vi "Teleop.vi"(10 "Match Info":T1={"Autonomous Elapsed Seconds"=0.0, "TeleOp Elapsed Seconds"=0.0, "Disabled Elapsed Seconds"=0.0, "Visited Autonomous"=FALSE, "Visited TeleOp"=FALSE, "Visited Disabled"=FALSE, "Autonomous Settings"={"Autonomous Style"=enum."Independent", "VI Refnum"=refnum}}, 11 "Call Context":T2) -> ()   [LabVIEW 2020]
doc: "This VI is called for each TeleOp packet received from the DS where the robot is not disabled. It is often used to read from the joysticks and update I/O or to update setpoints for timed control loops. It should complete and return within 20 milliseconds or it may miss DS packets."
uses:
  <vilib>/Rock Robotics/WPI/DriverStation/WPI_DriverStationDerivedRobotMode.ctl
  <vilib>/Rock Robotics/WPI/DriverStation/WPI_DriverStationMatch Info.ctl
  <vilib>/Rock Robotics/WPI/ThirdParty/Phoenix-LabVIEW/Motor Controller/Controls/CTRE_Phoenix_MotorControl_ControlMode.ctl
  <vilib>/Rock Robotics/WPI/Solenoid/WPI_SolenoidValue.ctl
  <vilib>/Rock Robotics/WPI/Utilities/WPI_GetSetVariantRefNum.vi
  <vilib>/Rock Robotics/Network Tables/NT Write Boolean Array.vi
  <vilib>/Rock Robotics/Network Tables/NT Write Numeric Array.vi
  <vilib>/Rock Robotics/Network Tables/NT Read Boolean.vi
  <vilib>/Rock Robotics/WPI/Solenoid/WPI_SolenoidSetEnum.vi
  Lime.vi
  <vilib>/Rock Robotics/WPI/RobotDrive/WPI_RobotDriveMecanumDrive_Cartesian.vi
panel:
  in  "Numeric":dbl=-0.7 format="%#_13g"
  in  "Auger Speed":dbl=-0.8
  out "Present Text":string
  in  "Total Time":dbl=0.9 format="%#_13g"
  in  "Time Low":dbl=0.6 format="%#_13g"
  in  "Slowmode Speed":dbl=0.33
  out "Compressor Running":bool
  out "Enabled":bool
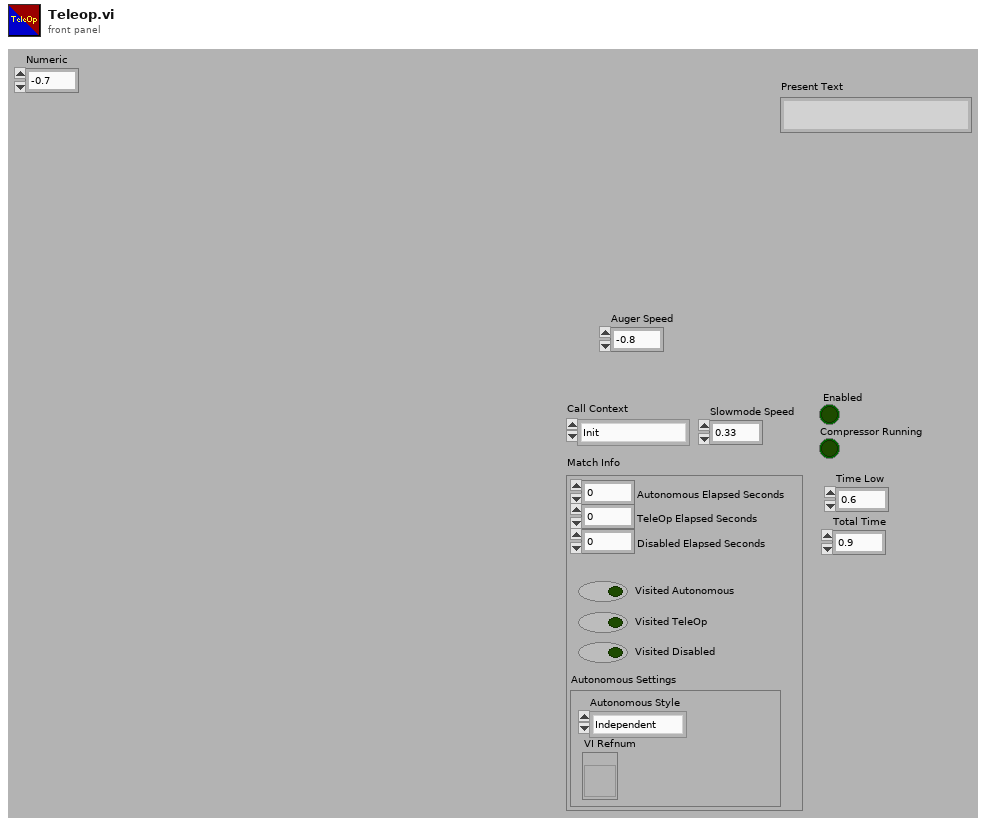
[diagram p1: front panel]
types:
  T1 = typedef "WPI_DriverStationMatch Info.ctl" = cluster{"Autonomous Elapsed Seconds":dbl, "TeleOp Elapsed Seconds":dbl, "Disabled Elapsed Seconds":dbl, "Visited Autonomous":bool, "Visited TeleOp":bool, "Visited Disabled":bool, "Autonomous Settings":cluster{"Autonomous Style":enum16{"Iterative", "Independent"}, "VI Refnum":refnum<vi>}}
  T2 = typedef "WPI_DriverStationDerivedRobotMode.ctl" = enum16{"Init", "Execute", "Stop"}
  T3 = typedef "CTRE_Phoenix_MotorControl_ControlMode.ctl" = u16
  T4 = typedef "WPI_JoystickDevRef.ctl" = cluster{"Device":T5}
  T5 = typedef "WPI_JoystickDeviceEnum.ctl" = enum16{"USB 0", "USB 1", "USB 2", "USB 3", "USB 4", "USB 5"}
  T6 = typedef "WPI_CompressorDevRef.ctl" = cluster{"DevStatus":errorcluster, "Pneumatics Control Module":u8}
  T7 = typedef "WPI_MotorControlDeviceRef.ctl" = cluster{"DeviceStatus":errorcluster, "Type":T8, "PWM":cluster{"PWM Channel":T9, "DeadBand":T10}, "CAN":cluster{"Device Number":u8, "SetOutput VI Ref":variant, "GetOutput VI Ref":variant, "Enable VI Ref":variant, "Disable VI Ref":variant, "Data":variant}, "Invert":bool, "DIO PWM":cluster{"PWM \"Enable\" Channel":T9, "DIOChannel":T11, "PWM Rate":dbl}}
  T8 = typedef "WPI_MotorControlType.ctl" = enum16{"PWM", "CAN", "DIO PWM"}
  T9 = typedef "FPGA_DIOPWMChannel.ctl" = enum8{"PWM 0", "PWM 1", "PWM 2", "PWM 3", "PWM 4", "PWM 5", "PWM 6", "PWM 7", "PWM 8", "PWM 9", "PWM MXP 0", "PWM MXP 1", "PWM MXP 2", "PWM MXP 3", "PWM MXP 4", "PWM MXP 5", "PWM MXP 6", "PWM MXP 7", "PWM MXP 8", "PWM MXP 9", "Invalid"}
  T10 = typedef "WPI_PWMDeadband.ctl" = cluster{"Name":string, "maxPositivePwm":i32, "minPositivePwm":i32, "centerPwm":i32, "maxNegativePwm":i32, "minNegativePwm":i32, "angularRange":u16}
  T11 = typedef "FPGA_DIOChannel.ctl" = enum8{"DIO 0", "DIO 1", "DIO 2", "DIO 3", "DIO 4", "DIO 5", "DIO 6", "DIO 7", "DIO 8", "DIO 9", "DIO MXP 0", "DIO MXP 1", "DIO MXP 2", "DIO MXP 3", "DIO MXP 4", "DIO MXP 5", "DIO MXP 6", "DIO MXP 7", "DIO MXP 8", "DIO MXP 9", "DIO MXP 10", "DIO MXP 11", "DIO MXP 12", "DIO MXP 13", "DIO MXP 14", "DIO MXP 15", "SPI Port CS1", "SPI Port CS2", "SPI Port CS3", "SPI Port MISO", "SPI Port MOSI", "Invalid"}
  T12 = typedef "WPI_RobotDriveDevRef.ctl" = cluster{"DevStatus":errorcluster, "Motors[]":T7[], "Square Inputs":bool, "Max Output":dbl}
  T13 = typedef "WPI_DigitalInputDevRef.ctl" = cluster{"DevStatus":errorcluster, "DIO Channel":T11}
  T14 = typedef "WPI_SolenoidValue.ctl" = enum16{"Off", "On", "Forward", "Reverse"}
  T15 = typedef "WPI_SolenoidDevRef.ctl" = cluster{"DevStatus":errorcluster, "Pneumatics Control Module":u8, "Forward Solenoid Channel":T16, "Reverse Solenoid Channel":T16}
  T16 = typedef "WPI_SolenoidChannel.ctl" = enum8{"Solenoid 0", "Solenoid 1", "Solenoid 2", "Solenoid 3", "Solenoid 4", "Solenoid 5", "Solenoid 6", "Solenoid 7", "Solenoid 8", "Solenoid 9", "Solenoid 10", "Solenoid 11", "Solenoid 12", "Solenoid 13", "Solenoid 14", "Solenoid 15", "Invalid"}
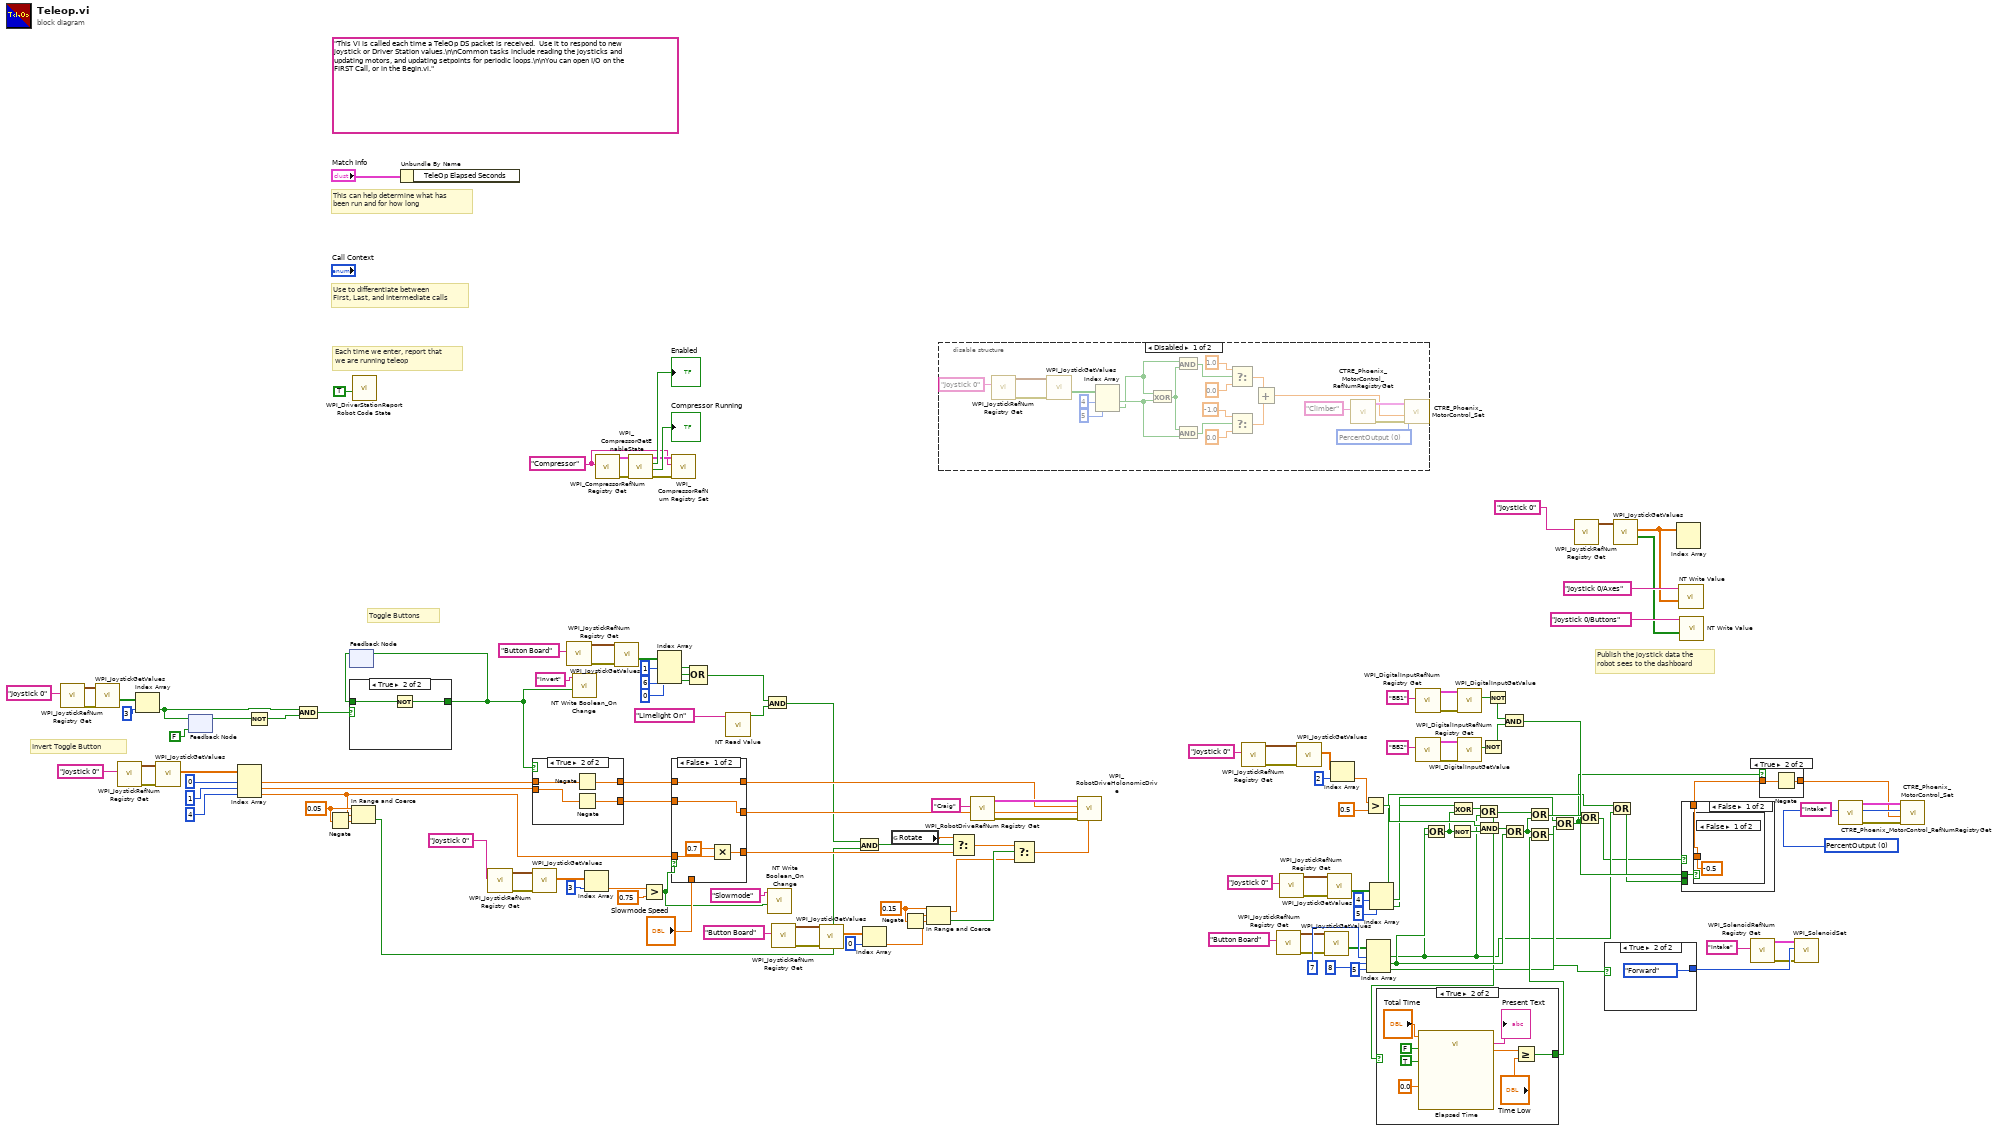
[diagram p0: block diagram]
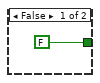
[diagram p3: hidden frame]
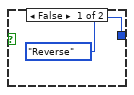
[diagram p4: hidden frame]
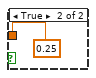
[diagram p5: hidden frame]
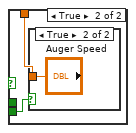
[diagram p6: hidden frame]
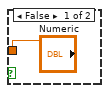
[diagram p7: hidden frame]
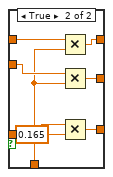
[diagram p8: hidden frame]
diagram:
  w4 = 0.15 ("upper limit")
  w15 = 0.05 ("upper limit")
  w54 = T3 0 items=["PercentOutput"=0, "Position"=1, "Velocity"=2, "Current"=3, "Follower"=5, "MotionProfile"=6, "MotionMagic"=7, "MotionProfileArc"=10, "Disabled"=15] ("Control Mode")
  w132 = "Compressor" ("refnum name")
  (unwired) "This VI is called each time a TeleOp DS packet is received.  Use it to respond to new joystick or Driver Station values.\n\nCommon tasks include reading the joysticks and updating motors, and updating setpoints for periodic loops.\n\nYou can open I/O on the FIRST Call, or in the Begin.vi."
  # "Invert Toggle Button"
  # "Toggle Buttons"
  # "Publish the joystick data the\nrobot sees to the dashboard"
  # "Each time we enter, report that\nwe are running teleop"
  # "Use to differentiate between\nFirst, Last, and Intermediate calls"
  # "This can help determine what has\nbeen run and for how long"
  n1 = call <vilib>:"WPI_JoystickRefNum Registry Get.vi"("refnum name"="Joystick 0") -> ("error out"=w121:errorcluster, "JoystickDevRef"=w110:T4)  [unwired: 9 in]
  n2 = call <vilib>:"WPI_JoystickGetValues.vi"("error in (no error)"=w121, "JoystickDevRef"=w110) -> ("Buttons"=w118:bool[])  [unwired: 5 in, 4 out]
  n3 = call <vilib>:"WPI_JoystickRefNum Registry Get.vi"("refnum name"="Joystick 0") -> ("error out"=w128:errorcluster, "JoystickDevRef"=w129:T4)  [unwired: 9 in]
  n4 = Index Array(array=w118, index=3) -> (element=w112:bool)
  n5 = call <vilib>:"WPI_JoystickGetValues.vi"("error in (no error)"=w128, "JoystickDevRef"=w129) -> ("Axes"=w125:dbl[])  [unwired: 5 in, 4 out]
  n6 = feedback #1(FALSE) -> (w114:bool)
  n7 = feedback-in #1(w112) -> ()
  n8 = Index Array(array=w125, index #1=0 ("index"), index #2=1 ("index"), index #3=4 ("index")) -> (element #1=w111:dbl, element #2=w98:dbl, element #3=w12:dbl)
  n9 = Not(x=w114) -> (.not. x?=w115:bool)
  n10 = And(x=w112, y=w115) -> (x .and. y?=w116:bool)
  n11 = Negate(x=w15) -> (-x=w16:dbl)
  n12 = feedback #2() -> (w117:bool)  [unwired: 1 in]
  n13 = case shown="True" w116 {
    tunnel: w117 -> [w147 w149]
    tunnel: [w147 w148] -> w97
    frame False {
    }
    frame True {
      n14 = Not(x=w149) -> (.not. x?=w148:bool)
    }
  }
  n15 = feedback-in #2(w97) -> ()
  n16 = In Range and Coerce(upper limit=w15, x=w12, lower limit=w16) -> (In Range?=w13:bool)  [unwired: 1 out]
  n17 = call <vilib>:"WPI_DriverStationReport Robot Code State.vi"("TeleOp"=TRUE ("Autonomous")) -> ()  [unwired: 10 in, 1 out]
  n18 = Unbundle By Name("Match Info") -> ()  [unwired: 1 out]
  n19 = call <vilib>:"WPI_JoystickRefNum Registry Get.vi"("refnum name"="Joystick 0") -> ("error out"=w104:errorcluster, "JoystickDevRef"=w107:T4)  [unwired: 9 in]
  n20 = case shown="True" w97 {
    tunnel: [w151 w152] -> w109
    tunnel: w111 -> [w151 w153]
    tunnel: [w150 w154] -> w108
    tunnel: w98 -> [w150 w155]
    frame False {
    }
    frame True {
      n21 = Negate(x=w153) -> (-x=w152:dbl)
      n22 = Negate(x=w155) -> (-x=w154:dbl)
    }
  }
  n23 = call <vilib>:"WPI_JoystickGetValues.vi"("error in (no error)"=w104, "JoystickDevRef"=w107) -> ("Axes"=w103:dbl[])  [unwired: 5 in, 4 out]
  n24 = call <vilib>:"WPI_JoystickRefNum Registry Get.vi"("refnum name"="Button Board") -> ("error out"=w92:errorcluster, "JoystickDevRef"=w90:T4)  [unwired: 9 in]
  n25 = call "NT Write Boolean_On Change.vi"("Boolean"=w97, "Name"="Invert") -> ()  [unwired: 9 in, 1 out]
  n26 = Index Array(array=w103, index=3) -> (element=w102:dbl)
  n27 = call <vilib>:"WPI_CompressorRefNum Registry Get.vi"("refnum name"=w132) -> ("error out"=w136:errorcluster, "CompressorDevRef"=w135:T6)  [unwired: 9 in]
  n28 = call <vilib>:"WPI_JoystickGetValues.vi"("error in (no error)"=w92, "JoystickDevRef"=w90) -> ("Buttons"=w91:bool[])  [unwired: 5 in, 4 out]
  n29 = call <vilib>:"WPI_CompressorGetEnableState.vi"("error in (no error)"=w136, "CompressorDevRef"=w135) -> ("error out"=w133:errorcluster, "Compressor Running"=→"Compressor Running":bool, "Enabled"=→"Enabled":bool, "CompressorDevRef"=w134:T6)  [unwired: 3 in, 3 out]
  n30 = Greater?(x=w102, y=0.75) -> (0:w94:bool)
  n31 = Index Array(array=w91, index #1=1 ("index"), index #2=6 ("index"), index #3=0 ("index")) -> (element #1=w83:bool, element #2=w85:bool, element #3=w84:bool)
  n32 = call <vilib>:"WPI_CompressorRefNum Registry Set.vi"("error in (no error)"=w133, "refnum name"=w132, "CompressorDevRef"=w134) -> ()  [unwired: 7 in, 2 out]
  n33 = case shown="False" w94 {
    tunnel: w12 -> [w160 w168]
    tunnel: [w157 w167] -> w18
    tunnel: w109 -> [w159 w166]
    tunnel: [w159 w165] -> w100
    tunnel: w108 -> [w158 w164]
    tunnel: [w158 w163] -> w86
    tunnel: "Slowmode Speed" -> [_ w162]
    frame False {
      n34 = Multiply(x=0.7, y=w160) -> (x*y=w157:dbl)
    }
    frame True {
      n35 = Multiply(x=w166, y=w162) -> (x*y=w165:dbl)
      n36 = Multiply(x=w164, y=w162) -> (x*y=w163:dbl)
      n37 = Multiply(x=w168, y=0.165) -> (x*y=w167:dbl)
    }
  }
  n38 = Compound Arithmetic op=OR(w83, w85, w84) -> (w80:bool)
  n39 = call-poly <vilib>:"NT Read Value.vi"("Name"="Limelight On") -> ("Boolean"=w82:bool)  [unwired: 9 in, 1 out]
  n40 = And(x=w80, y=w82) -> (x .and. y?=w20:bool)
  n41 = call "NT Write Boolean_On Change.vi"("Boolean"=w94, "Name"="Slowmode") -> ()  [unwired: 9 in, 1 out]
  n42 = call <vilib>:"WPI_JoystickRefNum Registry Get.vi"("refnum name"="Button Board") -> ("error out"=w9:errorcluster, "JoystickDevRef"=w10:T4)  [unwired: 9 in]
  n43 = call <vilib>:"WPI_JoystickGetValues.vi"("error in (no error)"=w9, "JoystickDevRef"=w10) -> ("Axes"=w7:dbl[])  [unwired: 5 in, 4 out]
  n44 = And(x=w20, y=w13) -> (x .and. y?=w14:bool)
  n45 = Index Array(array=w7, index=0) -> (element=w3:dbl)
  n46 = global read "Lime.vi" "Rotate"() -> (w19:dbl)
  n47 = Negate(x=w4) -> (-x=w6:dbl)
  n48 = In Range and Coerce(upper limit=w4, x=w3, lower limit=w6) -> (coerced(x)=w1:dbl, In Range?=w5:bool)
  n49 = disable-structure shown="Disabled" {
    frame Disabled {
      w189 = T3 0 items=["PercentOutput"=0, "Position"=1, "Velocity"=2, "Current"=3, "Follower"=5, "MotionProfile"=6, "MotionMagic"=7, "MotionProfileArc"=10, "Disabled"=15] ("Control Mode")
      n50 = call <vilib>:"WPI_JoystickRefNum Registry Get.vi"("refnum name"="Joystick 0") -> ("error out"=w185:errorcluster, "JoystickDevRef"=w186:T4)  [unwired: 9 in]
      n51 = call <vilib>:"WPI_JoystickGetValues.vi"("error in (no error)"=w185, "JoystickDevRef"=w186) -> ("Buttons"=w183:bool[])  [unwired: 5 in, 4 out]
      n52 = Index Array(array=w183, index #1=4 ("index"), index #2=5 ("index")) -> (element #1=w171:bool, element #2=w170:bool)
      n53 = Exclusive Or(1:w171, 2:w170) -> (0:w174:bool)
      n54 = And(x=w170, y=w174) -> (x .and. y?=w176:bool)
      n55 = And(x=w174, y=w171) -> (x .and. y?=w175:bool)
      n56 = Select(t=1.0, s=w176, f=0.0) -> (s? t:f=w172:dbl)
      n57 = Select(t=-1.0, s=w175, f=0.0) -> (s? t:f=w173:dbl)
      n58 = Add(x=w172, y=w173) -> (x+y=w169:dbl)
      n59 = call <vilib>:"CTRE_Phoenix_MotorControl_RefNumRegistryGet.vi"("refnum name"="Climber") -> ("error out"=w190:errorcluster, "PhoenixMotorControlDevRef"=w188:T7)  [unwired: 9 in]
      n60 = call <vilib>:"CTRE_Phoenix_MotorControl_Set.vi"("error in (no error)"=w190, "Output"=w169, "Control Mode"=w189, "PhoenixMotorControlDevRef"=w188) -> ()  [unwired: 6 in, 2 out]
    }
    frame Enabled {
    }
  }
  n61 = Select(t=w19, s=w14, f=w18) -> (s? t:f=w17:dbl)
  n62 = call <vilib>:"WPI_RobotDriveRefNum Registry Get.vi"("refnum name"="Craig") -> ("error out"=w130:errorcluster, "RobotDriveDevRef"=w131:T12)  [unwired: 9 in]
  n63 = Select(t=w17, s=w5, f=w1) -> (s? t:f=w2:dbl)
  n64 = call-poly <vilib>:"WPI_RobotDriveHolonomicDrive.vi"("Rotation"=w2, "error in (no error)"=w130, "Y"=w86, "X"=w100, "RobotDriveDevRef"=w131) -> ()  [unwired: 4 in, 3 out]
  n65 = call <vilib>:"WPI_JoystickRefNum Registry Get.vi"("refnum name"="Joystick 0") -> ("error out"=w59:errorcluster, "JoystickDevRef"=w58:T4)  [unwired: 9 in]
  n66 = call <vilib>:"WPI_JoystickRefNum Registry Get.vi"("refnum name"="Button Board") -> ("error out"=w42:errorcluster, "JoystickDevRef"=w40:T4)  [unwired: 9 in]
  n67 = call <vilib>:"WPI_JoystickRefNum Registry Get.vi"("refnum name"="Joystick 0") -> ("error out"=w65:errorcluster, "JoystickDevRef"=w67:T4)  [unwired: 9 in]
  n68 = call <vilib>:"WPI_JoystickGetValues.vi"("error in (no error)"=w59, "JoystickDevRef"=w58) -> ("Axes"=w60:dbl[])  [unwired: 5 in, 4 out]
  n69 = call <vilib>:"WPI_JoystickGetValues.vi"("error in (no error)"=w42, "JoystickDevRef"=w40) -> ("Buttons"=w41:bool[])  [unwired: 5 in, 4 out]
  n70 = call <vilib>:"WPI_JoystickGetValues.vi"("error in (no error)"=w65, "JoystickDevRef"=w67) -> ("Buttons"=w66:bool[])  [unwired: 5 in, 4 out]
  n71 = Index Array(array=w60, index=2) -> (element=w61:dbl)
  n72 = Greater?(x=w61, y=0.5) -> (0:w35:bool)
  n73 = Index Array(array=w41, index #1=7 ("index"), index #2=8 ("index"), index #3=5 ("index")) -> (element #1=w29:bool, element #2=w36:bool, element #3=w21:bool)
  n74 = Index Array(array=w66, index #1=4 ("index"), index #2=5 ("index")) -> (element #1=w30:bool, element #2=w24:bool)
  n75 = call <vilib>:"WPI_DigitalInputRefNum Registry Get.vi"("refnum name"="BB1") -> ("error out"=w79:errorcluster, "DigitalInputDevRef"=w78:T13)  [unwired: 9 in]
  n76 = call <vilib>:"WPI_DigitalInputRefNum Registry Get.vi"("refnum name"="BB2") -> ("error out"=w76:errorcluster, "DigitalInputDevRef"=w75:T13)  [unwired: 9 in]
  n77 = Or(x=w29, y=w36) -> (x .or. y?=w32:bool)
  n78 = Not(x=w32) -> (.not. x?=w33:bool)
  n79 = Exclusive Or(1:w32, 2:w30) -> (0:w38:bool)
  n80 = call <vilib>:"WPI_DigitalInputGetValue.vi"("error in (no error)"=w79, "DigitalInputDevRef"=w78) -> ("Value"=w73:bool)  [unwired: 7 in, 2 out]
  n81 = call <vilib>:"WPI_DigitalInputGetValue.vi"("error in (no error)"=w76, "DigitalInputDevRef"=w75) -> ("Value"=w72:bool)  [unwired: 7 in, 2 out]
  n82 = Or(x=w38, y=w29) -> (x .or. y?=w31:bool)
  n83 = case shown="True" w31 {
    tunnel: [FALSE w192] -> w46
    frame False {
    }
    frame True {
      n84 = call "Elapsed Time"("Time Target (s)"="Total Time", "Reset"=FALSE, "Auto Reset"=TRUE, "Set Start Time (s)"=0.0) -> ("Present Text"=→"Present Text":string, "Elapsed Time (s)"=w194:dbl)  [unwired: 8 in, 6 out]
      n85 = Greater Or Equal?(x=w194, y="Time Low") -> (x >= y?=w192:bool)
    }
  }
  n86 = And(x=w35, y=w33) -> (x .and. y?=w34:bool)
  n87 = Not(x=w72) -> (.not. x?=w70:bool)
  n88 = Not(x=w73) -> (.not. x?=w71:bool)
  n89 = And(x=w71, y=w70) -> (x .and. y?=w48:bool)
  n90 = Or(x=w34, y=w36) -> (x .or. y?=w37:bool)
  n91 = Or(x=w31, y=w37) -> (x .or. y?=w69:bool)
  n92 = Or(x=w37, y=w46) -> (x .or. y?=w47:bool)
  n93 = Or(x=w24, y=w21) -> (x .or. y?=w22:bool)
  n94 = call <vilib>:"WPI_JoystickRefNum Registry Get.vi"("refnum name"="Joystick 0") -> ("JoystickDevRef"=w144:T4)  [unwired: 1 in, 9 out]
  n95 = Or(x=w69, y=w22) -> (x .or. y?=w25:bool)
  n96 = case shown="True" w47 {
    tunnel: [WPI_SolenoidValue."Reverse" ("Value") WPI_SolenoidValue."Forward" ("Value")] -> w68
    frame False {
    }
    frame True {
    }
  }
  n97 = Or(x=w30, y=w29) -> (x .or. y?=w28:bool)
  n98 = call <vilib>:"WPI_JoystickGetValues.vi"("JoystickDevRef"=w144) -> ("Buttons"=w139:bool[], "Axes"=w140:dbl[])  [unwired: 6 in, 3 out]
  n99 = Index Array(array=w140) -> ()  [unwired: 2 in, 2 out]
  n100 = call-poly <vilib>:"NT Write Value.vi"("Numeric Array"=w140, "Name"="Joystick 0/Axes") -> ()  [unwired: 9 in, 1 out]
  n101 = call-poly <vilib>:"NT Write Value.vi"("Boolean Array"=w139, "Name"="Joystick 0/Buttons") -> ()  [unwired: 9 in, 1 out]
  n102 = case shown="False" w25 {
    tunnel: [w203 w207] -> w64
    tunnel: w48 -> [w202 _]
    tunnel: w28 -> [_ w206]
    frame False {
      n103 = case shown="False" w202 {
        tunnel: [-0.5 0.25] -> w203
        frame False {
        }
        frame True {
        }
      }
    }
    frame True {
      n104 = case shown="True" w206 {
        tunnel: ["Numeric" "Auger Speed"] -> w207
        frame False {
        }
        frame True {
        }
      }
    }
  }
  n105 = call <vilib>:"WPI_SolenoidRefNum Registry Get.vi"("refnum name"="Intake") -> ("error out"=w57:errorcluster, "SolenoidDevRef"=w56:T15)  [unwired: 9 in]
  n106 = case shown="True" w22 {
    tunnel: w64 -> [w210 w212]
    tunnel: [w210 w211] -> w26
    frame False {
    }
    frame True {
      n107 = Negate(x=w212) -> (-x=w211:dbl)
    }
  }
  n108 = call-poly <vilib>:"WPI_SolenoidSet.vi"("error in (no error)"=w57, "Value"=w68, "SolenoidDevRef"=w56) -> ()  [unwired: 7 in, 2 out]
  n109 = call <vilib>:"CTRE_Phoenix_MotorControl_RefNumRegistryGet.vi"("refnum name"="Intake") -> ("error out"=w63:errorcluster, "PhoenixMotorControlDevRef"=w62:T7)  [unwired: 9 in]
  n110 = call <vilib>:"CTRE_Phoenix_MotorControl_Set.vi"("error in (no error)"=w63, "Output"=w26, "Control Mode"=w54, "PhoenixMotorControlDevRef"=w62) -> ()  [unwired: 6 in, 2 out]
